vi "Core Action.vi"(8 "error in (no error)":errorcluster, 10 "SECS-II Class":refnum<class "SECS-II Class.lvclass">, 11 "19-Equipment Process Program Uploading in":refnum<class "19-Equipment Process Program Uploading.lvclass">) -> (0 "error out":errorcluster, 2 "SECS-II Class Out":refnum<class "SECS-II Class.lvclass">, 3 "19-Equipment Process Program Uploading out":refnum<class "19-Equipment Process Program Uploading.lvclass">)   [LabVIEW 2020, in "SECS Scenarios.lvlib" / "19-Equipment Process Program Uploading.lvclass"]
uses:
  19-Equipment Process Program Uploading.lvclass
  D:/Dropbox/SECS/SECS_GEM v1.1.0/Com/SECS Scenarios/Scenarios Class/Scenarios Class.lvclass
  SECS Communication/SECS-II Class/SECS-II Class.lvclass
  SECS Communication/S7 Message Class/S7 Message Class.lvclass
  D:/Dropbox/SECS/SECS_GEM v1.1.0/Com/SECS Communication/SECS-II Class/SECS-II Class.lvclass
  Scenarios Class/Reply State.ctl
  Scenarios Class/Scenarios Class.lvclass/Scenarios Class.ctl
  SECS Communication/S7 Message Class/S7F26.ctl
  SECS Communication/SECS-II Class/Format Code.ctl
  Scenarios Class/Write Reply State.vi
  Scenarios Class/Read HSMS Class.vi
  SECS Communication/SECS Data Class/Get ECID Data.vi
  SECS Communication/SECS-II Class/Variant To Data_ASCII.vi
  SECS Communication/HSMS Class/HSMS Class.lvclass
  Scenarios Class/Scenarios Class.lvclass
  SECS Communication/SECS Data Class/SECS Data Class.lvclass
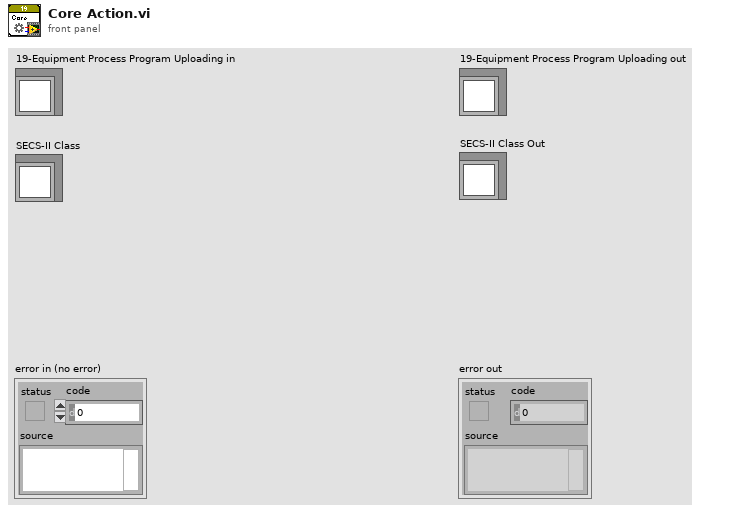
[diagram p1: front panel]
types:
  T1 = typedef "SECS Scenarios.lvlib/Scenarios Class.lvclass/Reply State.ctl" = enum16{"OK", "Illegal Data", "Unknown Stream", "Unknown Function", "Off-Line", "T3 Timeout", "Inner-Timeout"}
  T2 = typedef "SECS Communication.lvlib/S7 Message Class.lvclass/S7F26.ctl" = cluster{"PPID":string, "MDLN":string, "SOFTREV":string, "Parameter":cluster{"CCODE":string, "PPARM":cluster{"Format Code":T3, "Value":variant}[]}[]}
  T3 = typedef "SECS Communication.lvlib/SECS-II Class.lvclass/Format Code.ctl" = enum16{"L", "A", "B", "Boolean", "J", "I1", "I2", "I4", "I8", "U1", "U2", "U4", "U8", "F4", "F8", "Char"}
  T4 = cluster{"CCODE":string, "PPARM":cluster{"Format Code":T3, "Value":variant}[]}[]
  T5 = typedef "SECS Communication.lvlib/SECS Data Class.lvclass/ECID Data.ctl" = cluster{"ECID":u32, "Name":string, "Description":string, "Format Code":T3, "Unit":string, "Max":dbl, "Min":dbl, "Default":string, "Source":string, "Data":variant}
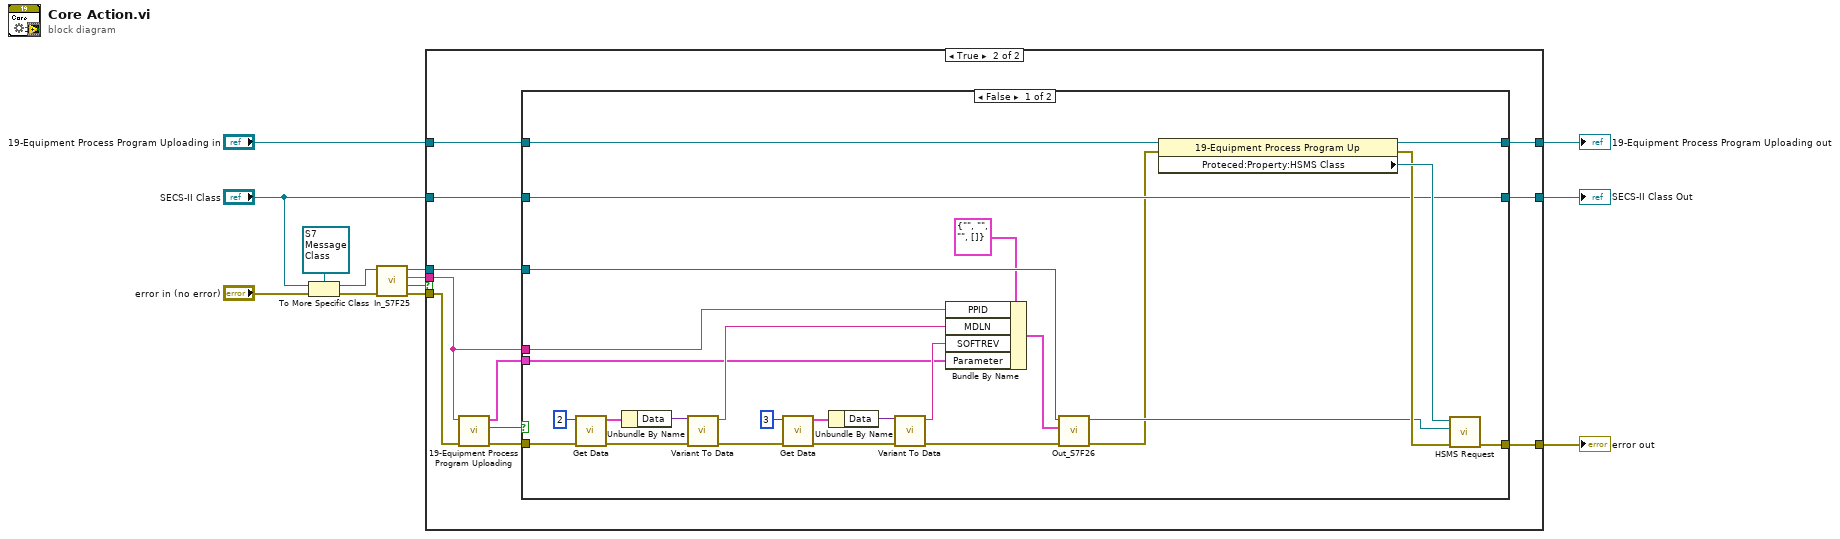
[diagram p0: block diagram]
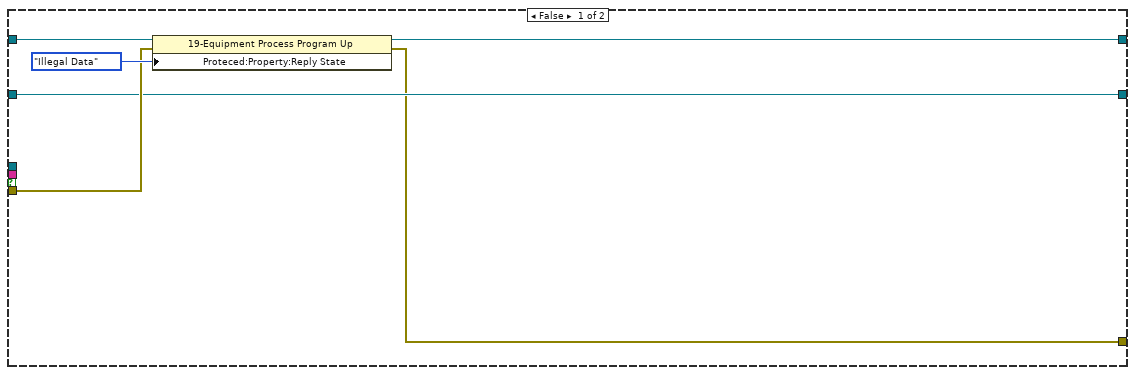
[diagram p2: hidden frame]
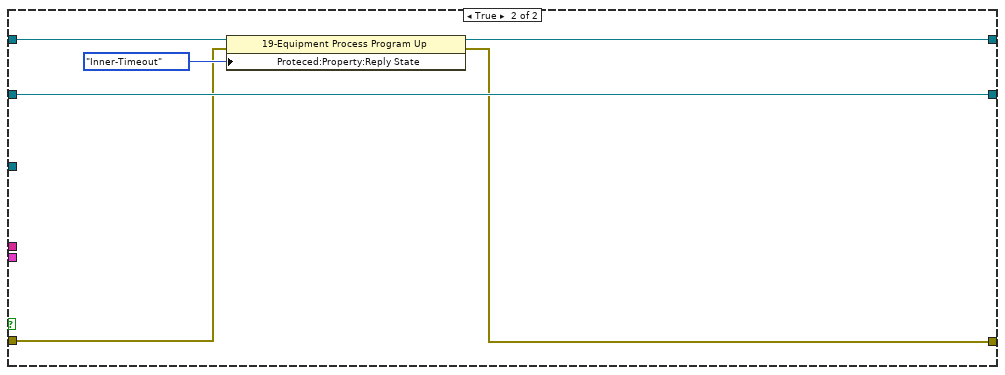
[diagram p3: hidden frame]
diagram:
  n1 = To More Specific Class(target class=refnum<class "S7 Message Class.lvclass"> refnum ("S7 Message Class in"), reference="SECS-II Class", error in="error in (no error)") -> (specific class reference=w11:refnum<class "S7 Message Class.lvclass">, error out=w12:errorcluster)
  n2 = call "In_S7F25.vi"("error in (no error)"=w12, "S7 Message Class in"=w11) -> ("error out"=w10:errorcluster, "OK?"=w1:bool, "PPID"=w6:string, "S7 Message Class out"=w9:refnum<class "S7 Message Class.lvclass">)  [unwired: 6 in]
  n3 = case shown="True" w1 {
    tunnel: w10 -> [w17 w30]
    tunnel: w9 -> [_ w29]
    tunnel: "19-Equipment Process Program Uploading in" -> [w19 w28]
    tunnel: w6 -> [_ w25]
    tunnel: [w15 w23] -> w5
    tunnel: [w14 w22] -> w4
    tunnel: "SECS-II Class" -> [w16 w21]
    tunnel: [w16 w20] -> w2
    frame False {
      n4 = property class="19-Equipment Process Program Up"(reference=w19, error in=w17, "Proteced:Property:Reply State"=Reply_State."Illegal Data" ("Reply State")) -> (reference out=w15:refnum<class "19-Equipment Process Program Uploading.lvclass">, error out=w14:errorcluster)
    }
    frame True {
      n5 = call "19-Equipment Process Program Uploading.vi"("error in (no error)"=w30, "PPID"=w25) -> ("error out"=w27:errorcluster, "Timeout?"=w26:bool, "Parameter"=w24:T4)  [unwired: 7 in]
      n6 = case shown="False" w26 {
        tunnel: w28 -> [w56 w60]
        tunnel: w29 -> [w51 _]
        tunnel: [w53 w57] -> w22
        tunnel: [w52 w58] -> w23
        tunnel: w27 -> [w38 w59]
        tunnel: w25 -> [w48 _]
        tunnel: w24 -> [w32 _]
        tunnel: w21 -> [w33 w62]
        tunnel: [w33 w62] -> w20
        frame False {
          n7 = call-poly "Get Data.vi"("error in"=w38, "ECID"=u32 2) -> ("error out"=w46:errorcluster, "ECID Data"=w47:T5)  [unwired: 7 in, 1 out]
          n8 = Unbundle By Name(w47) -> ("Data"=w45:variant)
          n9 = call-poly "Variant To Data.vi"("error in (no error)"=w46, "Variant"=w45) -> ("error out"=w39:errorcluster, "Data"=w36:string)  [unwired: 7 in, 1 out]
          n10 = call-poly "Get Data.vi"("error in"=w39, "ECID"=u32 3) -> ("error out"=w41:errorcluster, "ECID Data"=w40:T5)  [unwired: 7 in, 1 out]
          n11 = Unbundle By Name(w40) -> ("Data"=w42:variant)
          n12 = call-poly "Variant To Data.vi"("error in (no error)"=w41, "Variant"=w42) -> ("error out"=w37:errorcluster, "Data"=w35:string)  [unwired: 7 in, 1 out]
          n13 = Bundle By Name(cluster=T2 {"PPID"="", "MDLN"="", "SOFTREV"="", "Parameter"=[]} ("S7F26"), "PPID"=w48, "MDLN"=w36, "SOFTREV"=w35, "Parameter"=w32) -> (w34:T2)
          n14 = call "Out_S7F26.vi"("error in (no error)"=w37, "S7F26"=w34, "S7 Message Class in"=w51) -> ("error out"=w31:errorcluster, "S7 Message Class out"=w50:refnum<class "S7 Message Class.lvclass">)  [unwired: 7 in]
          n15 = property class="19-Equipment Process Program Up"(reference=w56, error in=w31) -> (reference out=w52:refnum<class "19-Equipment Process Program Uploading.lvclass">, error out=w54:errorcluster, "Proteced:Property:HSMS Class"=w55:refnum<class "HSMS Class.lvclass">)
          n16 = call "HSMS Request.vi"("error in (no error)"=w54, "SECS-II Class In"=w50, "HSMS Class in"=w55) -> ("error out"=w53:errorcluster)  [unwired: 7 in, 1 out]
        }
        frame True {
          n17 = property class="19-Equipment Process Program Up"(reference=w60, error in=w59, "Proteced:Property:Reply State"=Reply_State."Inner-Timeout" ("Reply State")) -> (reference out=w58:refnum<class "19-Equipment Process Program Uploading.lvclass">, error out=w57:errorcluster)
        }
      }
    }
  }
  "error out" <- w4
  "19-Equipment Process Program Uploading out" <- w5
  "SECS-II Class Out" <- w2
